vi "Remove empty daily folders.vi"(8 "error in (no error)":errorcluster) -> (0 "error out":errorcluster)   [LabVIEW 2017]
uses:
  Global Variables/General Globals.vi
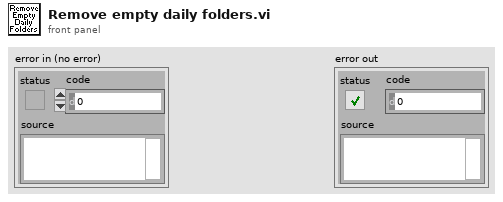
[diagram p1: front panel]
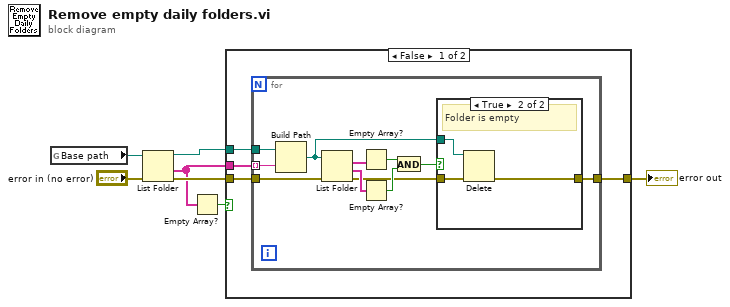
[diagram p0: block diagram]
diagram:
  n1 = global read "General Globals.vi" "Base path"() -> (w7:path)
  n2 = List Folder(path=w7, error in="error in (no error)") -> (path out=w5:path, folder names=w2:string[], error out=w4:errorcluster)  [unwired: 2 in, 1 out]
  n3 = Empty Array?(array=w2) -> (empty?=w1:bool)
  n4 = case shown="False" w1 {
    tunnel: w5 -> [w11 _]
    tunnel: w2 -> [w10 _]
    tunnel: w4 -> [w9 w27]
    tunnel: [w8 w27] -> w3
    frame False {
      n5 = for {
        tunnel: w11 -> [w22]
        tunnel: w10 -> [w21] mode=indexing
        tunnel: w9 -> [w15]
        tunnel: [w12] -> w8
        n6 = Build Path(base path=w22, name or relative path=w21) -> (appended path=w14:path)
        n7 = List Folder(path=w14, error in=w15) -> (filenames=w20:string[], folder names=w19:string[], error out=w13:errorcluster)  [unwired: 2 in, 1 out]
        n8 = Empty Array?(array=w20) -> (empty?=w18:bool)
        n9 = Empty Array?(array=w19) -> (empty?=w17:bool)
        n10 = And(x=w18, y=w17) -> (x .and. y?=w16:bool)
        n11 = case shown="True" w16 {
          tunnel: w14 -> [_ w26]
          tunnel: w13 -> [w23 w25]
          tunnel: [w23 w24] -> w12
          frame False {
            # "Folder is not empty"
          }
          frame True {
            # "Folder is empty"
            n12 = Delete(path (use dialog)=w26, error in=w25) -> (error out=w24:errorcluster)  [unwired: 3 in, 2 out]
          }
        }
      }
    }
    frame True {
    }
  }
  "error out" <- w3
